vi "MCL Release Handle.vi"(8 "error in (no error)":errorcluster, 11 "handle":i32) -> (0 "error out":errorcluster)   [LabVIEW 2014, in "Madlib.lvlib"]
doc: "MADLIB_API void MCL_ReleaseHandle(int handle);"
uses:
  Madlib.lvlib
  Program Files/Mad City Labs/TIRF-Lock/LabView 32-bit/Madlib.dll
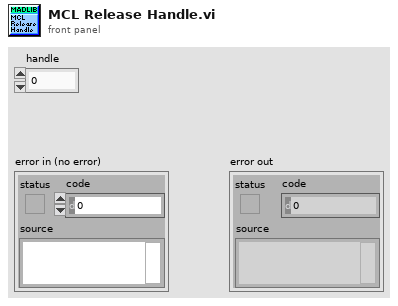
[diagram p1: front panel]
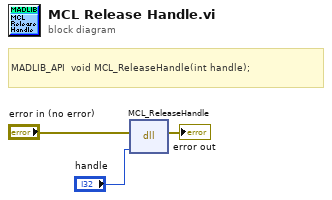
[diagram p0: block diagram]
diagram:
  # "MADLIB_API  void\tMCL_ReleaseHandle(int handle);"
  n1 = dll-call lib="C:/Program Files/Mad City Labs/TIRF-Lock/LabView 32-bit/Madlib.*" fn="MCL_ReleaseHandle"(error in="error in (no error)", "handle"="handle") -> (error out=→"error out":errorcluster)  [unwired: 4 in, 1 out]
